vi "Stop Core.vi"(10 "final error code":i32, 11 "Elevator Controller in":refnum<class "Sim User Console Actor.lvclass">) -> (3 "Elevator Controller out":refnum<class "Sim User Console Actor.lvclass">)   [LabVIEW 2019, in "Sim User Console Actor.lvlib" / "Sim User Console Actor.lvclass"]
doc: "(<B>Filename</B>: Actor Framework.lvlib:Actor.lvclass:Stop Core.vi)\n\nDefines what the actor does before it stops. Use the <B>final error code</B> input to determine whether the actor shut down in response to an error.\n\nBy default, this method passes the Stop message along to all auto-stop nested actors. A descendant class may override this method to define additional behavior, such as shutting down any processes the actor initiated in its override of the Actor Core method."
uses:
  Sim User Console Actor.lvclass
  Sim User Console Actor.lvclass/Sim User Console Actor.ctl
  User Console Actor/User Console Actor/User Console Actor.lvclass
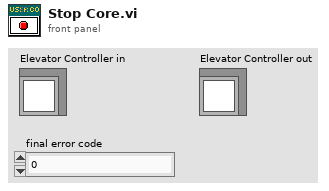
[diagram p1: front panel]
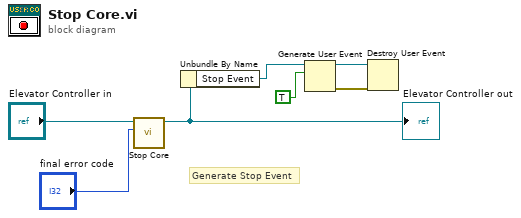
[diagram p0: block diagram]
diagram:
  # "Generate Stop Event"
  n1 = call-parent "Stop Core.vi"("final error code"="final error code", "Actor in"="Elevator Controller in") -> ("Actor out"=w5:refnum<class "Sim User Console Actor.lvclass">)  [unwired: 9 in]
  "Elevator Controller out" <- w5
  n2 = Unbundle By Name(w5) -> ("Stop Event"=w2:refnum<user-event>)
  n3 = Generate User Event(user event=w2, event data cluster=TRUE ("event data")) -> (user event out=w3:refnum<user-event>, error out=w4:errorcluster)  [unwired: 2 in]
  n4 = Destroy User Event(user event=w3, error in=w4) -> ()  [unwired: 1 out]
